vi "FeedbackDecode.vi"() -> ()   [LabVIEW 2020] (continued)
                n1302 = local read "NIPTime"() -> (w1168:dbl)
                n1303 = Concatenate Strings(w1160, w1180, w1179, w1178) -> (w1186:string)
                n1304 = Concatenate Strings("AutoPop:SS.EventID=" ("string"), w1164) -> (w1172:string)
                n1305 = local read "EventParamsFID"() -> (w1171:refnum<file>)
                n1306 = call-poly "FeedbackDecode_VariablesToString.vi"("Format"="%0.0f", "ValueIn"=w1168, "FieldName"="NIPTime" ("Key Word")) -> ("StringOut"=w1165:string)  [unwired: 4 in]
                n1307 = Concatenate Strings(w1172, ";", w1186, w1165) -> (w1170:string)
                n1308 = call "FeedbackDecode_WriteTextEOL.vi"("text"=w1170, "refnum in"=w1171) -> ()  [unwired: 8 in, 2 out]
                n1309 = Bundle By Name(cluster=w1187, "EventStr"=w1170) -> (w1169:T5)
                n1310 = call "FeedbackDecode_MLComCtrl.vi"("DecodeClustIn"=w1169, "Mode"=T19."SendEvent") -> ()  [unwired: 6 in, 4 out]
              }
            }
          }
          event Value Change {
            n1311 = event-data() -> ()  [unwired: 1 in, 6 out]
            n1312 = local read "DecodeClust"() -> (w1208:T5)
            n1313 = Unbundle By Name(w1208) -> ("BadUEAElects"=w1200:dbl[], "BadEMGChans"=w1203:dbl[])
            n1314 = local read "LoopCnt"() -> (w1196:u64)
            n1315 = call-poly "FeedbackDecode_VariablesToString.vi"("ValueIn"=w1200, "FieldName"="BadUEAElects") -> ("StringOut"=w1202:string)  [unwired: 5 in]
            n1316 = call-poly "FeedbackDecode_VariablesToString.vi"("ValueIn"=w1203, "FieldName"="BadEMGChans") -> ("StringOut"=w1201:string)  [unwired: 5 in]
            n1317 = Format Into String(w1196) -> (resulting string=w1188:string)  [unwired: 3 in, 1 out]
            n1318 = local read "NIPTime"() -> (w1192:dbl)
            n1319 = Concatenate Strings(w1202, w1201) -> (w1206:string)
            n1320 = Concatenate Strings("SendBad:SS.EventID=" ("string"), w1188) -> (w1195:string)
            n1321 = local read "EventParamsFID"() -> (w1207:refnum<file>)
            n1322 = call-poly "FeedbackDecode_VariablesToString.vi"("Format"="%0.0f", "ValueIn"=w1192, "FieldName"="NIPTime" ("Key Word")) -> ("StringOut"=w1189:string)  [unwired: 4 in]
            n1323 = Concatenate Strings(w1195, ";", w1206, w1189) -> (w1194:string)
            n1324 = call "FeedbackDecode_WriteTextEOL.vi"("text"=w1194, "refnum in"=w1207) -> ()  [unwired: 8 in, 2 out]
            n1325 = Bundle By Name(cluster=w1208, "EventStr"=w1194) -> (w1193:T5)
            n1326 = call "FeedbackDecode_MLComCtrl.vi"("DecodeClustIn"=w1193, "Mode"=T19."SendEvent") -> ()  [unwired: 6 in, 4 out]
          }
          event Value Change {
            n1327 = event-data() -> ("NewVal"=w1212:bool)  [unwired: 1 in, 5 out]
            n1328 = Not(x=w1212) -> (.not. x?=w1211:bool)
            n1329 = local read "DecodeClust"() -> (w1213:T5)
            n1330 = Bundle By Name(cluster=w1213, "CtrlButtons.Stop"=w1211) -> (w1210:T5)
            n1331 = local write "DecodeClust"(w1210) -> ()
            n1332 = property on="Finished" class="Bool (strict)"("DisabledEnum"=T17."Enabled" ("Disabled"), "Blinking"=TRUE) -> ()  [unwired: 2 in, 2 out]
            n1333 = local write "LVTab"(enum32{"Decode", "Encode", "Video", "Database"}."Database" ("LVTab")) -> ()
          }
          event "Finished": Value Change {
            n1334 = event-data() -> ("NewVal"=w1218:bool)  [unwired: 1 in, 5 out]
            n1335 = global write "FeedbackDecode_Globals.vi" "FD_Stop"(w1218) -> ()
          }
          event Value Change {
            n1336 = event-data() -> ("NewVal"=w1219:bool)  [unwired: 1 in, 5 out]
            n1337 = case shown="True" w1219 {
              frame False {
                n1338 = local read "LoopCnt"() -> (w1229:u64)
                n1339 = local read "NIPTime"() -> (w1225:dbl)
                n1340 = Format Into String(w1229) -> (resulting string=w1221:string)  [unwired: 3 in, 1 out]
                n1341 = local read "EventParamsFID"() -> (w1233:refnum<file>)
                n1342 = local read "DecodeClust"() -> (w1234:T5)
                n1343 = call-poly "FeedbackDecode_VariablesToString.vi"("Format"="%0.0f", "ValueIn"=w1225, "FieldName"="NIPTime" ("Key Word")) -> ("StringOut"=w1222:string)  [unwired: 4 in]
                n1344 = Concatenate Strings("DisableStartTrials:SS.EventID=" ("string"), w1221) -> (w1228:string)
                n1345 = Concatenate Strings(w1228, ";", w1222) -> (w1227:string)
                n1346 = call "FeedbackDecode_WriteTextEOL.vi"("text"=w1227, "refnum in"=w1233) -> ()  [unwired: 8 in, 2 out]
                n1347 = Bundle By Name(cluster=w1234, "EventStr"=w1227) -> (w1226:T5)
                n1348 = call "FeedbackDecode_MLComCtrl.vi"("DecodeClustIn"=w1226, "Mode"=T19."SendEvent") -> ()  [unwired: 6 in, 4 out]
              }
              frame True {
                n1349 = local read "LoopCnt"() -> (w1248:u64)
                n1350 = local read "NIPTime"() -> (w1239:dbl)
                n1351 = Format Into String(w1248) -> (resulting string=w1235:string)  [unwired: 3 in, 1 out]
                n1352 = local read "EventParamsFID"() -> (w1252:refnum<file>)
                n1353 = call-poly "FeedbackDecode_VariablesToString.vi"("Format"="%0.0f", "ValueIn"=w1239, "FieldName"="NIPTime" ("Key Word")) -> ("StringOut"=w1236:string)  [unwired: 4 in]
                n1354 = Concatenate Strings("EnableStartTrials:SS.EventID=" ("string"), w1235) -> (w1247:string)
                n1355 = Concatenate Strings(w1247, ";", w1236) -> (w1246:string)
                n1356 = local read "DecodeClust"() -> (w1253:T5)
                n1357 = call "FeedbackDecode_WriteTextEOL.vi"("text"=w1246, "refnum in"=w1252) -> ()  [unwired: 8 in, 2 out]
                n1358 = Initialize Array(0.0 ("element"), 2 ("dimension size"), 12 ("dimension size")) -> (w1241:dbl[][])
                n1359 = Bundle By Name(cluster=w1253, "EventStr"=w1246, "TrialCnt"=w1241) -> (w1245:T5)
                n1360 = local read "LoopCnt"() -> (w1255:u64)
                n1361 = local write "ResetCorr"(TRUE ("ResetCorr")) -> ()
                n1362 = call "FeedbackDecode_MLComCtrl.vi"("DecodeClustIn"=w1245, "Mode"=T19."SendEvent") -> ("DecodeClustOut"=w1240:T5)  [unwired: 6 in, 3 out]
                n1363 = local write "BaseCnt1"(w1255) -> ()
                n1364 = local write "DecodeClust"(w1240) -> ()
              }
            }
          }
          event Value Change {
            n1365 = event-data() -> ("CtlRef"=w1267:refnum<vi>)  [unwired: 1 in, 5 out]
            n1366 = property class="Ctl"(reference=w1267) -> ("Label.Text"=w1266:string)  [unwired: 1 in, 2 out]
            n1367 = case shown="\"ResetTrial\"" w1266 {
              frame "", Default {
              }
              frame "ResetTrial" {
                n1368 = local read "State"() -> (w1269:T16)
                n1369 = case shown="\"Acquire Start\", Default" w1269 {
                  frame "Initialize" {
                    n1370 = local read "DecodeClust"() -> (w1272:T5)
                    n1371 = Bundle By Name(cluster=w1272, "CtrlButtons.ResetTrial"=FALSE) -> (w1271:T5)
                    n1372 = local write "DecodeClust"(w1271) -> ()
                  }
                  frame "Acquire Start", Default {
                    n1373 = local read "NIPTime"() -> (w1277:dbl)
                    n1374 = local read "LoopCnt"() -> (w1281:u64)
                    n1375 = call-poly "FeedbackDecode_VariablesToString.vi"("Format"="%0.0f", "ValueIn"=w1277, "FieldName"="NIPTime" ("Key Word")) -> ("StringOut"=w1274:string)  [unwired: 4 in]
                    n1376 = Format Into String(w1281) -> (resulting string=w1273:string)  [unwired: 3 in, 1 out]
                    n1377 = local read "EventParamsFID"() -> (w1285:refnum<file>)
                    n1378 = local read "DecodeClust"() -> (w1286:T5)
                    n1379 = Concatenate Strings("ResetTrial:SS.EventID=" ("string"), w1273) -> (w1280:string)
                    n1380 = Concatenate Strings(w1280, ";", w1274) -> (w1279:string)
                    n1381 = call "FeedbackDecode_WriteTextEOL.vi"("text"=w1279, "refnum in"=w1285) -> ()  [unwired: 8 in, 2 out]
                    n1382 = Bundle By Name(cluster=w1286, "EventStr"=w1279) -> (w1278:T5)
                    n1383 = call "FeedbackDecode_MLComCtrl.vi"("DecodeClustIn"=w1278, "Mode"=T19."SendEvent") -> ()  [unwired: 6 in, 4 out]
                  }
                }
              }
            }
            n1384 = local read "MvntBuilder"() -> (w1258:T6)
            n1385 = Unbundle By Name(w1258) -> ("Mode"=w1265:enum16{"Selected", "Block", "Random"}, "NTrials"=w1262:dbl, "MvntList"=w1261:T24)
            n1386 = property on="MvntList" class="Arr (strict)"() -> ("Index Values"=w1259:u32[])  [unwired: 2 in, 2 out]
            n1387 = Array Size(array=w1261) -> (size(s)=w1260:i32)
            n1388 = Index Array(array=w1259) -> (element=w1263:u32)  [unwired: 1 in]
            n1389 = call "FeedbackDecode_GenRandBlockIdxs2.vi"("Mode"=w1265, "Reset"=TRUE, "NumTrials"=w1262, "NumIdxs"=w1260, "CurrIdx"=w1263) -> ("Perc"=w1257:dbl)  [unwired: 1 out]
            n1390 = Bundle By Name(cluster=w1258, "PercTrials"=w1257) -> (w1256:T6)
            n1391 = local write "MvntBuilder"(w1256) -> ()
          }
          event Value Change {
            n1392 = event-data() -> ("NewVal"=w1287:bool)  [unwired: 1 in, 5 out]
            n1393 = case shown="True" w1287 {
              frame False {
                n1394 = local read "LoopCnt"() -> (w1299:u64)
                n1395 = local read "NIPTime"() -> (w1293:dbl)
                n1396 = Format Into String(w1299) -> (resulting string=w1289:string)  [unwired: 3 in, 1 out]
                n1397 = call-poly "FeedbackDecode_VariablesToString.vi"("Format"="%0.0f", "ValueIn"=w1293, "FieldName"="NIPTime" ("Key Word")) -> ("StringOut"=w1290:string)  [unwired: 4 in]
                n1398 = Concatenate Strings("DisableHideSpheres:SS.EventID=" ("string"), w1289) -> (w1298:string)
                n1399 = local read "EventParamsFID"() -> (w1296:refnum<file>)
                n1400 = local read "DecodeClust"() -> (w1302:T5)
                n1401 = Concatenate Strings(w1298, ";SS.HideSpheres=0;" ("EventStr"), w1290) -> (w1295:string)
                n1402 = call "FeedbackDecode_WriteTextEOL.vi"("text"=w1295, "refnum in"=w1296) -> ()  [unwired: 8 in, 2 out]
                n1403 = Bundle By Name(cluster=w1302, "EventStr"=w1295) -> (w1294:T5)
                n1404 = call "FeedbackDecode_MLComCtrl.vi"("DecodeClustIn"=w1294, "Mode"=T19."SendEvent") -> ()  [unwired: 6 in, 4 out]
              }
              frame True {
                n1405 = local read "LoopCnt"() -> (w1313:u64)
                n1406 = local read "NIPTime"() -> (w1307:dbl)
                n1407 = Format Into String(w1313) -> (resulting string=w1303:string)  [unwired: 3 in, 1 out]
                n1408 = Concatenate Strings("EnableHideSpheres:SS.EventID=" ("string"), w1303) -> (w1312:string)
                n1409 = call-poly "FeedbackDecode_VariablesToString.vi"("Format"="%0.0f", "ValueIn"=w1307, "FieldName"="NIPTime" ("Key Word")) -> ("StringOut"=w1304:string)  [unwired: 4 in]
                n1410 = local read "EventParamsFID"() -> (w1310:refnum<file>)
                n1411 = local read "DecodeClust"() -> (w1316:T5)
                n1412 = Concatenate Strings(w1312, ";SS.HideSpheres=1;" ("EventStr"), w1304) -> (w1309:string)
                n1413 = call "FeedbackDecode_WriteTextEOL.vi"("text"=w1309, "refnum in"=w1310) -> ()  [unwired: 8 in, 2 out]
                n1414 = Bundle By Name(cluster=w1316, "EventStr"=w1309) -> (w1308:T5)
                n1415 = call "FeedbackDecode_MLComCtrl.vi"("DecodeClustIn"=w1308, "Mode"=T19."SendEvent") -> ()  [unwired: 6 in, 4 out]
              }
            }
          }
          event Value Change {
            n1416 = event-data() -> ("NewVal"=w1318:T44)  [unwired: 1 in, 5 out]
            n1417 = Format Into String(w1318) -> (resulting string=w1317:string)  [unwired: 3 in, 1 out]
            n1418 = local read "LoopCnt"() -> (w1327:u64)
            n1419 = call-poly "FeedbackDecode_VariablesToString.vi"("ValueIn"=w1317, "FieldName"="KalmanType") -> ("StringOut"=w1334:string)  [unwired: 5 in]
            n1420 = local read "NIPTime"() -> (w1323:dbl)
            n1421 = Format Into String(w1327) -> (resulting string=w1319:string)  [unwired: 3 in, 1 out]
            n1422 = local read "EventParamsFID"() -> (w1331:refnum<file>)
            n1423 = local read "DecodeClust"() -> (w1332:T5)
            n1424 = Concatenate Strings("ChangeKalmanType:SS.EventID=" ("string"), w1319) -> (w1326:string)
            n1425 = call-poly "FeedbackDecode_VariablesToString.vi"("Format"="%0.0f", "ValueIn"=w1323, "FieldName"="NIPTime" ("Key Word")) -> ("StringOut"=w1320:string)  [unwired: 4 in]
            n1426 = Concatenate Strings(w1326, ";", w1334, w1320) -> (w1325:string)
            n1427 = call "FeedbackDecode_WriteTextEOL.vi"("text"=w1325, "refnum in"=w1331) -> ()  [unwired: 8 in, 2 out]
            n1428 = Bundle By Name(cluster=w1332, "EventStr"=w1325) -> (w1324:T5)
            n1429 = call "FeedbackDecode_MLComCtrl.vi"("DecodeClustIn"=w1324, "Mode"=T19."SendEvent") -> ()  [unwired: 6 in, 4 out]
          }
          event Value Change {
            n1430 = event-data() -> ()  [unwired: 1 in, 6 out]
            n1431 = call "Load NN"("prompt"="select a .mat file that contains the trained NN") -> ("selected path"=w1338:path)  [unwired: 11 in, 3 out]
            n1432 = Path To String(path=w1338) -> (string=w1337:string)
            n1433 = local read "LoopCnt"() -> (w1347:u64)
            n1434 = call-poly "FeedbackDecode_VariablesToString.vi"("ValueIn"=w1337, "FieldName"="NN.path") -> ("StringOut"=w1354:string)  [unwired: 5 in]
            n1435 = local read "NIPTime"() -> (w1343:dbl)
            n1436 = Format Into String(w1347) -> (resulting string=w1339:string)  [unwired: 3 in, 1 out]
            n1437 = local read "EventParamsFID"() -> (w1351:refnum<file>)
            n1438 = Concatenate Strings("LoadNN:SS.EventID=" ("string"), w1339) -> (w1346:string)
            n1439 = call-poly "FeedbackDecode_VariablesToString.vi"("Format"="%0.0f", "ValueIn"=w1343, "FieldName"="NIPTime" ("Key Word")) -> ("StringOut"=w1340:string)  [unwired: 4 in]
            n1440 = Concatenate Strings(w1346, ";", w1354, w1340) -> (w1345:string)
            n1441 = local read "DecodeClust"() -> (w1352:T5)
            n1442 = call "FeedbackDecode_WriteTextEOL.vi"("text"=w1345, "refnum in"=w1351) -> ()  [unwired: 8 in, 2 out]
            n1443 = Bundle By Name(cluster=w1352, "EventStr"=w1345) -> (w1344:T5)
            n1444 = call "FeedbackDecode_MLComCtrl.vi"("DecodeClustIn"=w1344, "Mode"=T19."SendEvent") -> ()  [unwired: 6 in, 4 out]
          }
          event "CalibrateTASKA": Value Change {
            n1445 = event-data() -> ()  [unwired: 1 in, 6 out]
            n1446 = local read "LoopCnt"() -> (w1364:u64)
            n1447 = local read "NIPTime"() -> (w1360:dbl)
            n1448 = Format Into String(w1364) -> (resulting string=w1356:string)  [unwired: 3 in, 1 out]
            n1449 = local read "EventParamsFID"() -> (w1368:refnum<file>)
            n1450 = Concatenate Strings("CalibrateTASKA:SS.EventID=" ("string"), w1356) -> (w1363:string)
            n1451 = call-poly "FeedbackDecode_VariablesToString.vi"("Format"="%0.0f", "ValueIn"=w1360, "FieldName"="NIPTime" ("Key Word")) -> ("StringOut"=w1357:string)  [unwired: 4 in]
            n1452 = Concatenate Strings(w1363, ";", w1357) -> (w1362:string)
            n1453 = local read "DecodeClust"() -> (w1369:T5)
            n1454 = call "FeedbackDecode_WriteTextEOL.vi"("text"=w1362, "refnum in"=w1368) -> ()  [unwired: 8 in, 2 out]
            n1455 = Bundle By Name(cluster=w1369, "EventStr"=w1362) -> (w1361:T5)
            n1456 = call "FeedbackDecode_MLComCtrl.vi"("DecodeClustIn"=w1361, "Mode"=T19."SendEvent") -> ()  [unwired: 6 in, 4 out]
          }
          event "Reset Calibration": Value Change {
            n1457 = event-data() -> ()  [unwired: 1 in, 6 out]
            n1458 = local read "LoopCnt"() -> (w1379:u64)
            n1459 = local read "NIPTime"() -> (w1375:dbl)
            n1460 = Format Into String(w1379) -> (resulting string=w1371:string)  [unwired: 3 in, 1 out]
            n1461 = local read "EventParamsFID"() -> (w1383:refnum<file>)
            n1462 = Concatenate Strings("CalibrateTASKAreset:SS.EventID=" ("string"), w1371) -> (w1378:string)
            n1463 = call-poly "FeedbackDecode_VariablesToString.vi"("Format"="%0.0f", "ValueIn"=w1375, "FieldName"="NIPTime" ("Key Word")) -> ("StringOut"=w1372:string)  [unwired: 4 in]
            n1464 = Concatenate Strings(w1378, ";", w1372) -> (w1377:string)
            n1465 = local read "DecodeClust"() -> (w1384:T5)
            n1466 = call "FeedbackDecode_WriteTextEOL.vi"("text"=w1377, "refnum in"=w1383) -> ()  [unwired: 8 in, 2 out]
            n1467 = Bundle By Name(cluster=w1384, "EventStr"=w1377) -> (w1376:T5)
            n1468 = call "FeedbackDecode_MLComCtrl.vi"("DecodeClustIn"=w1376, "Mode"=T19."SendEvent") -> ()  [unwired: 6 in, 4 out]
          }
          event "LoadCyberGlove": Value Change {
            n1469 = event-data() -> ()  [unwired: 1 in, 6 out]
            n1470 = call "Load NN2"("prompt"="select a .mat file that contains the cyberglove calibration") -> ("selected path"=w1388:path)  [unwired: 11 in, 3 out]
            n1471 = Path To String(path=w1388) -> (string=w1387:string)
            n1472 = local read "LoopCnt"() -> (w1397:u64)
            n1473 = call-poly "FeedbackDecode_VariablesToString.vi"("ValueIn"=w1387, "FieldName"="CyberGlove.Calibration") -> ("StringOut"=w1404:string)  [unwired: 5 in]
            n1474 = local read "NIPTime"() -> (w1393:dbl)
            n1475 = Format Into String(w1397) -> (resulting string=w1389:string)  [unwired: 3 in, 1 out]
            n1476 = local read "EventParamsFID"() -> (w1401:refnum<file>)
            n1477 = local read "DecodeClust"() -> (w1402:T5)
            n1478 = Concatenate Strings("LoadCyberGlove:SS.EventID=" ("string"), w1389) -> (w1396:string)
            n1479 = call-poly "FeedbackDecode_VariablesToString.vi"("Format"="%0.0f", "ValueIn"=w1393, "FieldName"="NIPTime" ("Key Word")) -> ("StringOut"=w1390:string)  [unwired: 4 in]
            n1480 = Concatenate Strings(w1396, ";", w1404, w1390) -> (w1395:string)
            n1481 = call "FeedbackDecode_WriteTextEOL.vi"("text"=w1395, "refnum in"=w1401) -> ()  [unwired: 8 in, 2 out]
            n1482 = Bundle By Name(cluster=w1402, "EventStr"=w1395) -> (w1394:T5)
            n1483 = call "FeedbackDecode_MLComCtrl.vi"("DecodeClustIn"=w1394, "Mode"=T19."SendEvent") -> ()  [unwired: 6 in, 4 out]
          }
          event "Stim Thresholds": Value Change {
            # "convert from Newtons to 0 to 1 sensor value"
            n1484 = event-data() -> ("NewVal"=w1408:dbl[])  [unwired: 1 in, 5 out]
            n1485 = Divide(x=w1408, y=25.5) -> (x/y=w1409:dbl[])
            n1486 = local read "LoopCnt"() -> (w1418:u64)
            n1487 = call-poly "FeedbackDecode_VariablesToString.vi"("Format"="%0.6f", "ValueIn"=w1409, "FieldName"="DEKA.SensorThresholds") -> ("StringOut"=w1425:string)  [unwired: 4 in]
            n1488 = local read "NIPTime"() -> (w1414:dbl)
            n1489 = Format Into String(w1418) -> (resulting string=w1410:string)  [unwired: 3 in, 1 out]
            n1490 = local read "EventParamsFID"() -> (w1422:refnum<file>)
            n1491 = local read "DecodeClust"() -> (w1423:T5)
            n1492 = Concatenate Strings("UpdateSensorThresholds:SS.EventID=" ("string"), w1410) -> (w1417:string)
            n1493 = call-poly "FeedbackDecode_VariablesToString.vi"("Format"="%0.0f", "ValueIn"=w1414, "FieldName"="NIPTime" ("Key Word")) -> ("StringOut"=w1411:string)  [unwired: 4 in]
            n1494 = Concatenate Strings(w1417, ";", w1425, w1411) -> (w1416:string)
            n1495 = call "FeedbackDecode_WriteTextEOL.vi"("text"=w1416, "refnum in"=w1422) -> ()  [unwired: 8 in, 2 out]
            n1496 = Bundle By Name(cluster=w1423, "EventStr"=w1416) -> (w1415:T5)
            n1497 = call "FeedbackDecode_MLComCtrl.vi"("DecodeClustIn"=w1415, "Mode"=T19."SendEvent") -> ()  [unwired: 6 in, 4 out]
          }
          event Value Change {
            n1498 = event-data() -> ("NewVal"=w1433:string)  [unwired: 1 in, 5 out]
            n1499 = local read "LoopCnt"() -> (w1436:u64)
            n1500 = local read "NIPTime"() -> (w1431:dbl)
            n1501 = Format Into String(w1436) -> (resulting string=w1427:string)  [unwired: 3 in, 1 out]
            n1502 = local read "DecodeClust"() -> (w1441:T5)
            n1503 = Concatenate Strings("SS.LinkedDOF=" ("FieldName"), w1433, ";" ("string")) -> (w1444:string)
            n1504 = local read "EventParamsFID"() -> (w1440:refnum<file>)
            n1505 = Concatenate Strings("LinkDOF:SS.EventID=" ("string"), w1427) -> (w1435:string)
            n1506 = call-poly "FeedbackDecode_VariablesToString.vi"("Format"="%0.0f", "ValueIn"=w1431, "FieldName"="NIPTime" ("Key Word")) -> ("StringOut"=w1428:string)  [unwired: 4 in]
            n1507 = Concatenate Strings(w1435, ";", w1444, w1428) -> (w1434:string)
            n1508 = call "FeedbackDecode_WriteTextEOL.vi"("text"=w1434, "refnum in"=w1440) -> ()  [unwired: 8 in, 2 out]
            n1509 = Bundle By Name(cluster=w1441, "EventStr"=w1434) -> (w1432:T5)
            n1510 = call "FeedbackDecode_MLComCtrl.vi"("DecodeClustIn"=w1432, "Mode"=T19."SendEvent") -> ()  [unwired: 6 in, 4 out]
          }
          event Value Change {
            n1511 = event-data() -> ("NewVal"=w1452:enum16{"Standard", "Stepwise", "Gram"})  [unwired: 1 in, 5 out]
            n1512 = local read "LoopCnt"() -> (w1455:u64)
            n1513 = call-poly "FeedbackDecode_VariablesToString.vi"("Format"="%0.0f", "ValueIn"=w1452, "FieldName"="AutoPopType") -> ("StringOut"=w1463:string)  [unwired: 4 in]
            n1514 = local read "NIPTime"() -> (w1450:dbl)
            n1515 = Format Into String(w1455) -> (resulting string=w1446:string)  [unwired: 3 in, 1 out]
            n1516 = local read "EventParamsFID"() -> (w1459:refnum<file>)
            n1517 = local read "DecodeClust"() -> (w1460:T5)
            n1518 = Concatenate Strings("ChangeAutoPopType:SS.EventID=" ("string"), w1446) -> (w1454:string)
            n1519 = call-poly "FeedbackDecode_VariablesToString.vi"("Format"="%0.0f", "ValueIn"=w1450, "FieldName"="NIPTime" ("Key Word")) -> ("StringOut"=w1447:string)  [unwired: 4 in]
            n1520 = Concatenate Strings(w1454, ";", w1463, w1447) -> (w1453:string)
            n1521 = call "FeedbackDecode_WriteTextEOL.vi"("text"=w1453, "refnum in"=w1459) -> ()  [unwired: 8 in, 2 out]
            n1522 = Bundle By Name(cluster=w1460, "EventStr"=w1453) -> (w1451:T5)
            n1523 = call "FeedbackDecode_MLComCtrl.vi"("DecodeClustIn"=w1451, "Mode"=T19."SendEvent") -> ()  [unwired: 6 in, 4 out]
          }
          event Value Change {
            n1524 = event-data() -> ("NewVal"=w1466:enum16{"Standard", "NN"})  [unwired: 1 in, 5 out]
            n1525 = Format Into String(w1466) -> (resulting string=w1465:string)  [unwired: 3 in, 1 out]
            n1526 = local read "LoopCnt"() -> (w1475:u64)
            n1527 = call-poly "FeedbackDecode_VariablesToString.vi"("ValueIn"=w1465, "FieldName"="CARType") -> ("StringOut"=w1482:string)  [unwired: 5 in]
            n1528 = local read "NIPTime"() -> (w1471:dbl)
            n1529 = Format Into String(w1475) -> (resulting string=w1467:string)  [unwired: 3 in, 1 out]
            n1530 = local read "EventParamsFID"() -> (w1479:refnum<file>)
            n1531 = Concatenate Strings("ChangeCARType:SS.EventID=" ("string"), w1467) -> (w1474:string)
            n1532 = local read "DecodeClust"() -> (w1480:T5)
            n1533 = call-poly "FeedbackDecode_VariablesToString.vi"("Format"="%0.0f", "ValueIn"=w1471, "FieldName"="NIPTime" ("Key Word")) -> ("StringOut"=w1468:string)  [unwired: 4 in]
            n1534 = Concatenate Strings(w1474, ";", w1482, w1468) -> (w1473:string)
            n1535 = call "FeedbackDecode_WriteTextEOL.vi"("text"=w1473, "refnum in"=w1479) -> ()  [unwired: 8 in, 2 out]
            n1536 = Bundle By Name(cluster=w1480, "EventStr"=w1473) -> (w1472:T5)
            n1537 = call "FeedbackDecode_MLComCtrl.vi"("DecodeClustIn"=w1472, "Mode"=T19."SendEvent") -> ()  [unwired: 6 in, 4 out]
          }
          event Value Change {
            n1538 = event-data() -> ("NewVal"=w1486:bool)  [unwired: 1 in, 5 out]
            n1539 = Boolean To (0,1)(Boolean=w1486) -> (0, 1=w1485:i16)
            n1540 = local read "LoopCnt"() -> (w1495:u64)
            n1541 = call-poly "FeedbackDecode_VariablesToString.vi"("Format"="%0.0f", "ValueIn"=w1485, "FieldName"="LimitExt") -> ("StringOut"=w1502:string)  [unwired: 4 in]
            n1542 = local read "NIPTime"() -> (w1491:dbl)
            n1543 = Format Into String(w1495) -> (resulting string=w1487:string)  [unwired: 3 in, 1 out]
            n1544 = local read "DecodeClust"() -> (w1500:T5)
            n1545 = local read "EventParamsFID"() -> (w1499:refnum<file>)
            n1546 = Concatenate Strings("LimitExt:SS.EventID=" ("string"), w1487) -> (w1494:string)
            n1547 = call-poly "FeedbackDecode_VariablesToString.vi"("Format"="%0.0f", "ValueIn"=w1491, "FieldName"="NIPTime" ("Key Word")) -> ("StringOut"=w1488:string)  [unwired: 4 in]
            n1548 = Concatenate Strings(w1494, ";", w1502, w1488) -> (w1493:string)
            n1549 = call "FeedbackDecode_WriteTextEOL.vi"("text"=w1493, "refnum in"=w1499) -> ()  [unwired: 8 in, 2 out]
            n1550 = Bundle By Name(cluster=w1500, "EventStr"=w1493) -> (w1492:T5)
            n1551 = call "FeedbackDecode_MLComCtrl.vi"("DecodeClustIn"=w1492, "Mode"=T19."SendEvent") -> ()  [unwired: 6 in, 4 out]
          }
          event Value Change {
            n1552 = event-data() -> ("NewVal"=w1506:bool)  [unwired: 1 in, 5 out]
            n1553 = Boolean To (0,1)(Boolean=w1506) -> (0, 1=w1505:i16)
            n1554 = local read "LoopCnt"() -> (w1515:u64)
            n1555 = call-poly "FeedbackDecode_VariablesToString.vi"("Format"="%0.0f", "ValueIn"=w1505, "FieldName"="DynFlag") -> ("StringOut"=w1522:string)  [unwired: 4 in]
            n1556 = local read "NIPTime"() -> (w1511:dbl)
            n1557 = Format Into String(w1515) -> (resulting string=w1507:string)  [unwired: 3 in, 1 out]
            n1558 = local read "DecodeClust"() -> (w1520:T5)
            n1559 = local read "EventParamsFID"() -> (w1519:refnum<file>)
            n1560 = Concatenate Strings("DynFlag:SS.EventID=" ("string"), w1507) -> (w1514:string)
            n1561 = call-poly "FeedbackDecode_VariablesToString.vi"("Format"="%0.0f", "ValueIn"=w1511, "FieldName"="NIPTime" ("Key Word")) -> ("StringOut"=w1508:string)  [unwired: 4 in]
            n1562 = Concatenate Strings(w1514, ";", w1522, w1508) -> (w1513:string)
            n1563 = call "FeedbackDecode_WriteTextEOL.vi"("text"=w1513, "refnum in"=w1519) -> ()  [unwired: 8 in, 2 out]
            n1564 = Bundle By Name(cluster=w1520, "EventStr"=w1513) -> (w1512:T5)
            n1565 = call "FeedbackDecode_MLComCtrl.vi"("DecodeClustIn"=w1512, "Mode"=T19."SendEvent") -> ()  [unwired: 6 in, 4 out]
          }
          event Mouse Move {
            n1566 = event-data() -> ("Coords"=w1531:T45)  [unwired: 1 in, 3 out]
            n1567 = local read "HoverPicPos"() -> (w1529:T14)
            n1568 = call "FeedbackDecode_HoverElect.vi"("Border"=2.0, "PicPos"=w1529, "MousePos"=w1531, "Mode"=enum16{"Initialize", "Run"}."Run") -> ("Elect"=w1524:i32)  [unwired: 2 in, 1 out]
            n1569 = local read "DecodeClust"() -> (w1526:T5)
            n1570 = Bundle By Name(cluster=w1526, "HoverElect"=w1524) -> (w1525:T5)
            n1571 = local write "DecodeClust"(w1525) -> ()
          }
          event Value Change {
            # "Also updated CtrlMode and CtrlSpd"
            n1572 = event-data() -> ()  [unwired: 1 in, 6 out]
            n1573 = local read "DecodeClust"() -> (w1537:T5)
            n1574 = Unbundle By Name(w1537) -> ("KMvntClust"=w1538:T46)
            n1575 = call "FeedbackDecode_KalmanMvnts2Str.vi"("KMvntClust"=w1538) -> ("KMvntStr"=w1534:string)
            n1576 = Concatenate Strings("UpdateKGainThresh:" ("string"), w1534) -> (w1533:string)
            n1577 = Bundle By Name(cluster=w1537, "EventStr"=w1533) -> (w1532:T5)
            n1578 = call "FeedbackDecode_MLComCtrl.vi"("DecodeClustIn"=w1532, "Mode"=T19."SendEvent") -> ()  [unwired: 6 in, 4 out]
          }
          event Value Change {
            n1579 = event-data() -> ("NewVal"=w1541:bool)  [unwired: 1 in, 5 out]
            n1580 = case shown="True" w1541 {
              frame False {
              }
              frame True {
                n1581 = local read "DecodeClust"() -> (w1565:T5)
                n1582 = Unbundle By Name(w1565) -> ("ThreshMode"=w1543:T47, "ThreshVal"=w1560:dbl)
                n1583 = Format Into String(w1543) -> (resulting string=w1542:string)  [unwired: 3 in, 1 out]
                n1584 = local read "LoopCnt"() -> (w1554:u64)
                n1585 = call-poly "FeedbackDecode_VariablesToString.vi"("ValueIn"=w1542, "FieldName"="ThreshMode") -> ("StringOut"=w1562:string)  [unwired: 5 in]
                n1586 = call-poly "FeedbackDecode_VariablesToString.vi"("ValueIn"=w1560, "FieldName"="ThreshVal") -> ("StringOut"=w1559:string)  [unwired: 5 in]
                n1587 = local read "NIPTime"() -> (w1548:dbl)
                n1588 = Concatenate Strings(w1562, w1559) -> (w1564:string)
                n1589 = Format Into String(w1554) -> (resulting string=w1544:string)  [unwired: 3 in, 1 out]
                n1590 = local read "EventParamsFID"() -> (w1558:refnum<file>)
                n1591 = call-poly "FeedbackDecode_VariablesToString.vi"("Format"="%0.0f", "ValueIn"=w1548, "FieldName"="NIPTime" ("Key Word")) -> ("StringOut"=w1545:string)  [unwired: 4 in]
                n1592 = Concatenate Strings("UpdateThresh:SS.EventID=" ("string"), w1544) -> (w1553:string)
                n1593 = Concatenate Strings(w1553, ";", w1564, w1545) -> (w1552:string)
                n1594 = call "FeedbackDecode_WriteTextEOL.vi"("text"=w1552, "refnum in"=w1558) -> ()  [unwired: 8 in, 2 out]
                n1595 = Bundle By Name(cluster=w1565, "EventStr"=w1552, "ApplyThresh"=FALSE) -> (w1551:T5)
                n1596 = call "FeedbackDecode_MLComCtrl.vi"("DecodeClustIn"=w1551, "Mode"=T19."SendEvent") -> ("DecodeClustOut"=w1549:T5)  [unwired: 6 in, 3 out]
                n1597 = local write "DecodeClust"(w1549) -> ()
              }
            }
          }
          event Value Change {
            n1598 = event-data() -> ("NewVal"=w1570:dbl)  [unwired: 1 in, 5 out]
            n1599 = Divide(x=w1570, y=0.033) -> (x/y=w1566:dbl)
            n1600 = Multiply(x=2.0, y=w1566) -> (x*y=w1568:dbl)
            n1601 = property on="SelData" class="WFGraph (strict)"("XScale.Maximum"=w1568) -> ()  [unwired: 2 in, 2 out]
            n1602 = property on="SelRate" class="WFGraph (strict)"("XScale.Maximum"=w1566) -> ()  [unwired: 2 in, 2 out]
            n1603 = property on="SelKin" class="WFGraph (strict)"("XScale.Maximum"=w1566) -> ()  [unwired: 2 in, 2 out]
          }
          event Value Change {
            n1604 = event-data() -> ("NewVal"=w1573:bool)  [unwired: 1 in, 5 out]
            n1605 = case shown="True" w1573 {
              frame False {
              }
              frame True {
                n1606 = for {
                  N: 2 -> [_]
                  tunnel: [w1579] -> w1574 mode=indexing
                  n1607 = Initialize Array(FALSE, 100 ("dimension size")) -> (w1580:bool[])
                  n1608 = Array To Cluster(array=w1580) -> (cluster=w1579:T48)
                }
                n1609 = local read "DecodeClust"() -> (w1577:T5)
                n1610 = Bundle By Name(cluster=w1577, "ClearUEA"=FALSE ("CtrlButtons.ResetTrial"), "KUEAArray"=w1574) -> (w1576:T5)
                n1611 = local write "DecodeClust"(w1576) -> ()
              }
            }
          }
          event Value Change {
            n1612 = event-data() -> ("NewVal"=w1584:bool)  [unwired: 1 in, 5 out]
            n1613 = case shown="True" w1584 {
              frame False {
              }
              frame True {
                n1614 = for {
                  N: 2 -> [_]
                  tunnel: [w1590] -> w1585 mode=indexing
                  n1615 = Initialize Array(TRUE, 100 ("dimension size")) -> (w1591:bool[])
                  n1616 = Array To Cluster(array=w1591) -> (cluster=w1590:T48)
                }
                n1617 = local read "DecodeClust"() -> (w1588:T5)
                n1618 = Bundle By Name(cluster=w1588, "FillUEA"=FALSE ("CtrlButtons.ResetTrial"), "KUEAArray"=w1585) -> (w1587:T5)
                n1619 = local write "DecodeClust"(w1587) -> ()
              }
            }
          }
          event Value Change {
            n1620 = event-data() -> ("NewVal"=w1595:bool)  [unwired: 1 in, 5 out]
            n1621 = case shown="True" w1595 {
              frame False {
              }
              frame True {
                n1622 = Initialize Array(FALSE, 80 ("dimension size")) -> (w1601:bool[])
                n1623 = Array To Cluster(array=w1601) -> (cluster=w1597:T49)
                n1624 = local read "DecodeClust"() -> (w1600:T5)
                n1625 = Bundle By Name(cluster=w1600, "ClearEMG"=FALSE ("CtrlButtons.ResetTrial"), "KEMGClust"=w1597, "KEMGExtra"=dbl[] []) -> (w1599:T5)
                n1626 = local write "DecodeClust"(w1599) -> ()
              }
            }
          }
          event Value Change {
            n1627 = event-data() -> ("NewVal"=w1605:bool)  [unwired: 1 in, 5 out]
            n1628 = case shown="True" w1605 {
              frame False {
              }
              frame True {
                n1629 = Initialize Array(TRUE, 80 ("dimension size")) -> (w1610:bool[])
                n1630 = Array To Cluster(array=w1610) -> (cluster=w1606:T49)
                n1631 = local read "DecodeClust"() -> (w1607:T5)
                n1632 = Bundle By Name(cluster=w1607, "FillEMG"=FALSE ("CtrlButtons.ResetTrial"), "KEMGClust"=w1606) -> (w1608:T5)
                n1633 = local write "DecodeClust"(w1608) -> ()
              }
            }
          }
          event Value Change {
            n1634 = event-data() -> ()  [unwired: 1 in, 6 out]
            n1635 = local read "DecodeClust"() -> (w1628:T5)
            n1636 = Unbundle By Name(w1628) -> ("GainFill"=w1627:dbl, "ThreshFill"=w1626:dbl, "ModeFill"=w1617:T50, "SpdFill"=w1614:dbl)
            n1637 = Initialize Array(w1627, 12 ("dimension size"), 2 ("dimension size")) -> (w1632:dbl[][])
            n1638 = Initialize Array(w1626, 12 ("dimension size"), 2 ("dimension size")) -> (w1629:dbl[][])
            n1639 = Initialize Array(w1617, 12 ("dimension size")) -> (w1616:T43)
            n1640 = Initialize Array(w1614, 12 ("dimension size")) -> (w1613:dbl[])
            n1641 = Bundle By Name(cluster=w1628, "KMvntClust.KGain"=w1632, "KMvntClust.KThresh"=w1629, "KMvntClust.CtrlMode"=w1616, "KMvntClust.CtrlSpd"=w1613, "FillMvnts"=FALSE ("ClearKalman")) -> (w1619:T5)
            n1642 = Unbundle By Name(w1619) -> ("KMvntClust"=w1625:T46)
            n1643 = local write "DecodeClust"(w1619) -> ()
            n1644 = call "FeedbackDecode_KalmanMvnts2Str.vi"("KMvntClust"=w1625) -> ("KMvntStr"=w1622:string)
            n1645 = Concatenate Strings("UpdateKGainThresh:" ("string"), w1622) -> (w1621:string)
            n1646 = Bundle By Name(cluster=w1619, "EventStr"=w1621) -> (w1620:T5)
            n1647 = call "FeedbackDecode_MLComCtrl.vi"("DecodeClustIn"=w1620, "Mode"=T19."SendEvent") -> ()  [unwired: 6 in, 4 out]
          }
          event Value Change {
            n1648 = event-data() -> ("NewVal"=w1637:bool)  [unwired: 1 in, 5 out]
            n1649 = case shown="True" w1637 {
              frame False {
              }
              frame True {
                n1650 = Initialize Array(0.0 ("element"), 2 ("dimension size"), 12 ("dimension size")) -> (w1639:dbl[][])
                n1651 = local read "DecodeClust"() -> (w1642:T5)
                n1652 = Bundle By Name(cluster=w1642, "ClearTrials"=FALSE ("CtrlButtons.ResetTrial"), "TrialCnt"=w1639) -> (w1641:T5)
                n1653 = local write "DecodeClust"(w1641) -> ()
              }
            }
          }
          event Value Change {
            n1654 = event-data() -> ("NewVal"=w1652:dbl)  [unwired: 1 in, 5 out]
            n1655 = local read "LoopCnt"() -> (w1655:u64)
            n1656 = local read "NIPTime"() -> (w1650:dbl)
            n1657 = call-poly "FeedbackDecode_VariablesToString.vi"("ValueIn"=w1652, "FieldName"="Lag") -> ("StringOut"=w1662:string)  [unwired: 5 in]
            n1658 = local read "DecodeClust"() -> (w1660:T5)
            n1659 = Format Into String(w1655) -> (resulting string=w1646:string)  [unwired: 3 in, 1 out]
            n1660 = local read "EventParamsFID"() -> (w1659:refnum<file>)
            n1661 = call-poly "FeedbackDecode_VariablesToString.vi"("Format"="%0.0f", "ValueIn"=w1650, "FieldName"="NIPTime" ("Key Word")) -> ("StringOut"=w1647:string)  [unwired: 4 in]
            n1662 = Concatenate Strings("ChangeLag:SS.EventID=" ("string"), w1646) -> (w1654:string)
            n1663 = Concatenate Strings(w1654, ";", w1662, w1647) -> (w1653:string)
            n1664 = call "FeedbackDecode_WriteTextEOL.vi"("text"=w1653, "refnum in"=w1659) -> ()  [unwired: 8 in, 2 out]
            n1665 = Bundle By Name(cluster=w1660, "EventStr"=w1653) -> (w1651:T5)
            n1666 = call "FeedbackDecode_MLComCtrl.vi"("DecodeClustIn"=w1651, "Mode"=T19."SendEvent") -> ()  [unwired: 6 in, 4 out]
          }
          event Value Change {
            n1667 = event-data() -> ("NewVal"=w1670:dbl)  [unwired: 1 in, 5 out]
            n1668 = local read "LoopCnt"() -> (w1673:u64)
            n1669 = local read "NIPTime"() -> (w1668:dbl)
            n1670 = call-poly "FeedbackDecode_VariablesToString.vi"("ValueIn"=w1670, "FieldName"="KernelWidth") -> ("StringOut"=w1680:string)  [unwired: 5 in]
            n1671 = local read "DecodeClust"() -> (w1678:T5)
            n1672 = Format Into String(w1673) -> (resulting string=w1664:string)  [unwired: 3 in, 1 out]
            n1673 = local read "EventParamsFID"() -> (w1677:refnum<file>)
            n1674 = call-poly "FeedbackDecode_VariablesToString.vi"("Format"="%0.0f", "ValueIn"=w1668, "FieldName"="NIPTime" ("Key Word")) -> ("StringOut"=w1665:string)  [unwired: 4 in]
            n1675 = Concatenate Strings("ChangeKernel:SS.EventID=" ("string"), w1664) -> (w1672:string)
            n1676 = Concatenate Strings(w1672, ";", w1680, w1665) -> (w1671:string)
            n1677 = call "FeedbackDecode_WriteTextEOL.vi"("text"=w1671, "refnum in"=w1677) -> ()  [unwired: 8 in, 2 out]
            n1678 = Bundle By Name(cluster=w1678, "EventStr"=w1671) -> (w1669:T5)
            n1679 = call "FeedbackDecode_MLComCtrl.vi"("DecodeClustIn"=w1669, "Mode"=T19."SendEvent") -> ()  [unwired: 6 in, 4 out]
          }
          event Value Change {
            n1680 = event-data() -> ("NewVal"=w1688:dbl)  [unwired: 1 in, 5 out]
            n1681 = local read "LoopCnt"() -> (w1691:u64)
            n1682 = local read "NIPTime"() -> (w1686:dbl)
            n1683 = call-poly "FeedbackDecode_VariablesToString.vi"("ValueIn"=w1688, "FieldName"="TargRad") -> ("StringOut"=w1698:string)  [unwired: 5 in]
            n1684 = local read "DecodeClust"() -> (w1696:T5)
            n1685 = Format Into String(w1691) -> (resulting string=w1682:string)  [unwired: 3 in, 1 out]
            n1686 = local read "EventParamsFID"() -> (w1695:refnum<file>)
            n1687 = call-poly "FeedbackDecode_VariablesToString.vi"("Format"="%0.0f", "ValueIn"=w1686, "FieldName"="NIPTime" ("Key Word")) -> ("StringOut"=w1683:string)  [unwired: 4 in]
            n1688 = Concatenate Strings("ChangeTargRad:SS.EventID=" ("string"), w1682) -> (w1690:string)
            n1689 = Concatenate Strings(w1690, ";", w1698, w1683) -> (w1689:string)
            n1690 = call "FeedbackDecode_WriteTextEOL.vi"("text"=w1689, "refnum in"=w1695) -> ()  [unwired: 8 in, 2 out]
            n1691 = Bundle By Name(cluster=w1696, "EventStr"=w1689) -> (w1687:T5)
            n1692 = call "FeedbackDecode_MLComCtrl.vi"("DecodeClustIn"=w1687, "Mode"=T19."SendEvent") -> ()  [unwired: 6 in, 4 out]
          }
          event Value Change {
            n1693 = event-data() -> ("NewVal"=w1706:T37)  [unwired: 1 in, 5 out]
            n1694 = local read "LoopCnt"() -> (w1709:u64)
            n1695 = Format Into String(w1706) -> (resulting string=w1717:string)  [unwired: 3 in, 1 out]
            n1696 = local read "NIPTime"() -> (w1704:dbl)
            n1697 = local read "DecodeClust"() -> (w1714:T5)
            n1698 = Format Into String(w1709) -> (resulting string=w1700:string)  [unwired: 3 in, 1 out]
            n1699 = Concatenate Strings("SS.KinSrc='" ("string"), w1717, "';" ("string")) -> (w1718:string)
            n1700 = local read "EventParamsFID"() -> (w1713:refnum<file>)
            n1701 = call-poly "FeedbackDecode_VariablesToString.vi"("Format"="%0.0f", "ValueIn"=w1704, "FieldName"="NIPTime" ("Key Word")) -> ("StringOut"=w1701:string)  [unwired: 4 in]
            n1702 = Concatenate Strings("ChangeKinSrc:SS.EventID=" ("string"), w1700) -> (w1708:string)
            n1703 = Concatenate Strings(w1708, ";", w1718, w1701) -> (w1707:string)
            n1704 = call "FeedbackDecode_WriteTextEOL.vi"("text"=w1707, "refnum in"=w1713) -> ()  [unwired: 8 in, 2 out]
            n1705 = Bundle By Name(cluster=w1714, "EventStr"=w1707) -> (w1705:T5)
            n1706 = call "FeedbackDecode_MLComCtrl.vi"("DecodeClustIn"=w1705, "Mode"=T19."SendEvent") -> ()  [unwired: 6 in, 4 out]
          }
          event Value Change {
            n1707 = event-data() -> ("NewVal"=w1720:T23)  [unwired: 1 in, 5 out]
            n1708 = local read "LoopCnt"() -> (w1729:u64)
            n1709 = Format Into String(w1720) -> (resulting string=w1737:string)  [unwired: 3 in, 1 out]
            n1710 = local read "NIPTime"() -> (w1725:dbl)
            n1711 = local read "DecodeClust"() -> (w1734:T5)
            n1712 = Format Into String(w1729) -> (resulting string=w1721:string)  [unwired: 3 in, 1 out]
            n1713 = Concatenate Strings("SS.TestType='" ("string"), w1737, "';" ("string")) -> (w1738:string)
            n1714 = local read "EventParamsFID"() -> (w1733:refnum<file>)
            n1715 = call-poly "FeedbackDecode_VariablesToString.vi"("Format"="%0.0f", "ValueIn"=w1725, "FieldName"="NIPTime" ("Key Word")) -> ("StringOut"=w1722:string)  [unwired: 4 in]
            n1716 = Concatenate Strings("ChangeTestType:SS.EventID=" ("string"), w1721) -> (w1728:string)
            n1717 = Concatenate Strings(w1728, ";", w1738, w1722) -> (w1727:string)
            n1718 = call "FeedbackDecode_WriteTextEOL.vi"("text"=w1727, "refnum in"=w1733) -> ()  [unwired: 8 in, 2 out]
            n1719 = Bundle By Name(cluster=w1734, "EventStr"=w1727) -> (w1726:T5)
            n1720 = call "FeedbackDecode_MLComCtrl.vi"("DecodeClustIn"=w1726, "Mode"=T19."SendEvent") -> ()  [unwired: 6 in, 4 out]
          }
          event Value Change {
            n1721 = event-data() -> ("NewVal"=w1740:bool)  [unwired: 1 in, 5 out]
            n1722 = case shown="True" w1740 {
              frame False {
              }
              frame True {
                n1723 = local read "LoopCnt"() -> (w1753:u64)
                n1724 = local read "NIPTime"() -> (w1746:dbl)
                n1725 = Format Into String(w1753) -> (resulting string=w1742:string)  [unwired: 3 in, 1 out]
                n1726 = local read "EventParamsFID"() -> (w1757:refnum<file>)
                n1727 = call-poly "FeedbackDecode_VariablesToString.vi"("Format"="%0.0f", "ValueIn"=w1746, "FieldName"="NIPTime" ("Key Word")) -> ("StringOut"=w1743:string)  [unwired: 4 in]
                n1728 = Concatenate Strings("ResetVRE:SS.EventID=" ("string"), w1742) -> (w1752:string)
                n1729 = Concatenate Strings(w1752, ";", w1743) -> (w1751:string)
                n1730 = local read "DecodeClust"() -> (w1758:T5)
                n1731 = call "FeedbackDecode_WriteTextEOL.vi"("text"=w1751, "refnum in"=w1757) -> ()  [unwired: 8 in, 2 out]
                n1732 = Bundle By Name(cluster=w1758, "EventStr"=w1751, "CtrlButtons.ResetVRE"=FALSE ("ResetVRE")) -> (w1750:T5)
                n1733 = property on="StimMode" class="Enum (strict)"("Val(Sgnl)"=enum16{"Off", "Manual", "MSMS", "VRE"}."Off" ("Value (Signaling)")) -> ()  [unwired: 2 in, 2 out]
                n1734 = call "FeedbackDecode_MLComCtrl.vi"("DecodeClustIn"=w1750, "Mode"=T19."SendEvent") -> ("DecodeClustOut"=w1748:T5)  [unwired: 6 in, 3 out]
                n1735 = local write "DecodeClust"(w1748) -> ()
              }
            }
          }
          event Value Change {
            n1736 = event-data() -> ("NewVal"=w1759:bool)  [unwired: 1 in, 5 out]
            n1737 = case shown="True" w1759 {
              frame False {
              }
              frame True {
                n1738 = local read "LoopCnt"() -> (w1772:u64)
                n1739 = local read "NIPTime"() -> (w1765:dbl)
                n1740 = Format Into String(w1772) -> (resulting string=w1761:string)  [unwired: 3 in, 1 out]
                n1741 = local read "EventParamsFID"() -> (w1776:refnum<file>)
                n1742 = Concatenate Strings("StopVRE:SS.EventID=" ("string"), w1761) -> (w1771:string)
                n1743 = call-poly "FeedbackDecode_VariablesToString.vi"("Format"="%0.0f", "ValueIn"=w1765, "FieldName"="NIPTime" ("Key Word")) -> ("StringOut"=w1762:string)  [unwired: 4 in]
                n1744 = Concatenate Strings(w1771, ";", w1762) -> (w1770:string)
                n1745 = local read "DecodeClust"() -> (w1777:T5)
                n1746 = call "FeedbackDecode_WriteTextEOL.vi"("text"=w1770, "refnum in"=w1776) -> ()  [unwired: 8 in, 2 out]
                n1747 = Bundle By Name(cluster=w1777, "EventStr"=w1770, "CtrlButtons.StopVRE"=FALSE ("ResetVRE")) -> (w1769:T5)
                n1748 = property on="StimMode" class="Enum (strict)"("Val(Sgnl)"=enum16{"Off", "Manual", "MSMS", "VRE"}."Off" ("Value (Signaling)")) -> ()  [unwired: 2 in, 2 out]
                n1749 = call "FeedbackDecode_MLComCtrl.vi"("DecodeClustIn"=w1769, "Mode"=T19."SendEvent") -> ("DecodeClustOut"=w1767:T5)  [unwired: 6 in, 3 out]
                n1750 = local write "DecodeClust"(w1767) -> ()
              }
            }
          }
          event Value Change {
            n1751 = event-data() -> ("NewVal"=w1778:bool)  [unwired: 1 in, 5 out]
            n1752 = case shown="True" w1778 {
              frame False {
              }
              frame True {
                n1753 = local read "LoopCnt"() -> (w1790:u64)
                n1754 = local read "NIPTime"() -> (w1784:dbl)
                n1755 = Format Into String(w1790) -> (resulting string=w1780:string)  [unwired: 3 in, 1 out]
                n1756 = local read "EventParamsFID"() -> (w1794:refnum<file>)
                n1757 = Concatenate Strings("ConARD:SS.EventID=" ("string"), w1780) -> (w1789:string)
                n1758 = call-poly "FeedbackDecode_VariablesToString.vi"("Format"="%0.0f", "ValueIn"=w1784, "FieldName"="NIPTime" ("Key Word")) -> ("StringOut"=w1781:string)  [unwired: 4 in]
                n1759 = Concatenate Strings(w1789, ";", w1781) -> (w1788:string)
                n1760 = local read "DecodeClust"() -> (w1795:T5)
                n1761 = call "FeedbackDecode_WriteTextEOL.vi"("text"=w1788, "refnum in"=w1794) -> ()  [unwired: 8 in, 2 out]
                n1762 = Bundle By Name(cluster=w1795, "EventStr"=w1788, "CtrlButtons.ConARD"=FALSE ("ResetVRE")) -> (w1787:T5)
                n1763 = call "FeedbackDecode_MLComCtrl.vi"("DecodeClustIn"=w1787, "Mode"=T19."SendEvent") -> ("DecodeClustOut"=w1785:T5)  [unwired: 6 in, 3 out]
                n1764 = local write "DecodeClust"(w1785) -> ()
              }
            }
          }
          event Value Change {
            n1765 = event-data() -> ("NewVal"=w1797:bool)  [unwired: 1 in, 4 out]
            n1766 = case shown="True" w1797 {
              frame False {
              }
              frame True {
                n1767 = property on="MvntList" class="Arr (strict)"() -> ("Index Values"=w1801:u32[])  [unwired: 2 in, 2 out]
                n1768 = local read "MvntBuilder"() -> (w1805:T6)
                n1769 = Index Array(array=w1801) -> (element=w1806:u32)  [unwired: 1 in]
                n1770 = local read "DecodeClust"() -> (w1800:T5)
                n1771 = Bundle By Name(cluster=w1800, "CtrlButtons.StartTrials"=FALSE) -> (w1798:T5)
                n1772 = call "FeedbackDecode_SetMvntBuilder.vi"("MvntBuilderIn"=w1805, "MvntIdx"=w1806) -> ("MvntBuilderOut"=w1804:T6)  [unwired: 1 in]
                n1773 = Bundle By Name(cluster=w1804, "Set"=FALSE) -> (w1802:T6)
                n1774 = local write "MvntBuilder"(w1802) -> ()
                n1775 = local write "DecodeClust"(w1798) -> ()
              }
            }
          }
          event Value Change {
            n1776 = event-data() -> ("NewVal"=w1808:bool)  [unwired: 1 in, 4 out]
            n1777 = case shown="True" w1808 {
              frame False {
              }
              frame True {
                n1778 = local read "MvntBuilder"() -> (w1813:T6)
                n1779 = local read "DecodeClust"() -> (w1812:T5)
                n1780 = Bundle By Name(cluster=w1812, "CtrlButtons.StartTrials"=FALSE) -> (w1810:T5)
                n1781 = Bundle By Name(cluster=w1813, "MvntList"=T24 [], "Clear"=FALSE ("Set")) -> (w1814:T6)
                n1782 = local write "MvntBuilder"(w1814) -> ()
                n1783 = local write "DecodeClust"(w1810) -> ()
              }
            }
          }
          event Value Change {
            n1784 = event-data() -> ("NewVal"=w1817:bool)  [unwired: 1 in, 5 out]
            n1785 = case shown="True" w1817 {
              frame False {
              }
              frame True {
                n1786 = flat-sequence {
                  frame #0 {
                    n1787 = local read "MvntBuilder"() -> (w1821:T6)
                    n1788 = local read "DecodeClust"() -> (w1820:T5)
                    n1789 = Bundle By Name(cluster=w1820, "CtrlButtons.StartTrials"=FALSE) -> (w1818:T5)
                    n1790 = Bundle By Name(cluster=w1821, "Load"=FALSE ("Set")) -> (w1822:T6)
                    n1791 = local write "MvntBuilder"(w1822) -> ()
                    n1792 = local write "DecodeClust"(w1818) -> ()
                  }
                  frame #1 {
                    n1793 = local read "MvntBuilder"() -> (w1825:T6)
                    n1794 = call "FeedbackDecode_MvntListIO.vi"("MvntBuilderIn"=w1825, "Mode"=enum16{"Read", "Write"}."Read") -> ("MvntBuilderOut"=w1824:T6)  [unwired: 1 in]
                    n1795 = Unbundle By Name(w1824) -> ("MvntList"=w1827:T24)
                    n1796 = property on="MvntList" class="Arr (strict)"("Val(Sgnl)"=w1827) -> ()  [unwired: 2 in, 2 out]
                  }
                }
              }
            }
          }
          event Value Change {
            n1797 = event-data() -> ("NewVal"=w1828:bool)  [unwired: 1 in, 5 out]
            n1798 = case shown="True" w1828 {
              frame False {
              }
              frame True {
                n1799 = flat-sequence {
                  frame #0 {
                    n1800 = local read "MvntBuilder"() -> (w1833:T6)
                    n1801 = local read "DecodeClust"() -> (w1832:T5)
                    n1802 = Bundle By Name(cluster=w1832, "CtrlButtons.StartTrials"=FALSE) -> (w1830:T5)
                    n1803 = Bundle By Name(cluster=w1833, "Save"=FALSE ("Set")) -> (w1834:T6)
                    n1804 = local write "MvntBuilder"(w1834) -> ()
                    n1805 = local write "DecodeClust"(w1830) -> ()
                  }
                  frame #1 {
                    n1806 = local read "MvntBuilder"() -> (w1836:T6)
                    n1807 = call "FeedbackDecode_MvntListIO.vi"("MvntBuilderIn"=w1836, "Mode"=enum16{"Read", "Write"}."Write") -> ()  [unwired: 1 in, 1 out]
                  }
                }
              }
            }
          }
          event Value Change {
            n1808 = event-data() -> ("OldVal"=w1841:T24, "NewVal"=w1840:T24)  [unwired: 1 in, 4 out]
            n1809 = Array Size(array=w1841) -> (size(s)=w1842:i32)
            n1810 = Array Size(array=w1840) -> (size(s)=w1843:i32)
            n1811 = Not Equal?(x=w1842, y=w1843) -> (x != y?=w1839:bool)
            n1812 = case shown="True" w1839 {
              frame False {
              }
              frame True {
                n1813 = local read "MvntBuilder"() -> (w1846:T6)
                n1814 = local read "DecodeClust"() -> (w1856:T5)
                n1815 = Bundle By Name(cluster=w1856, "CtrlButtons.StartTrials"=FALSE) -> (w1854:T5)
                n1816 = Unbundle By Name(w1846) -> ("Mode"=w1853:enum16{"Selected", "Block", "Random"}, "NTrials"=w1850:dbl, "MvntList"=w1849:T24)
                n1817 = property on="MvntList" class="Arr (strict)"() -> ("Index Values"=w1847:u32[])  [unwired: 2 in, 2 out]
                n1818 = Array Size(array=w1849) -> (size(s)=w1848:i32)
                n1819 = Index Array(array=w1847) -> (element=w1851:u32)  [unwired: 1 in]
                n1820 = local write "DecodeClust"(w1854) -> ()
                n1821 = call "FeedbackDecode_GenRandBlockIdxs2.vi"("Mode"=w1853, "Reset"=TRUE, "NumTrials"=w1850, "NumIdxs"=w1848, "CurrIdx"=w1851) -> ("Perc"=w1845:dbl)  [unwired: 1 out]
                n1822 = Bundle By Name(cluster=w1846, "PercTrials"=w1845) -> (w1844:T6)
                n1823 = local write "MvntBuilder"(w1844) -> ()
              }
            }
          }
          event Value Change {
            n1824 = event-data() -> ("NewVal"=w1857:dbl)  [unwired: 1 in, 5 out]
            n1825 = local read "MSMSSphere"() -> (w1863:dbl[][])
            n1826 = Initialize Array(w1857, 6 ("dimension size")) -> (w1859:dbl[])
            n1827 = property on="TargRad" class="DigNum (strict)"("Val(Sgnl)"=w1857) -> ()  [unwired: 2 in, 2 out]
            n1828 = Replace Array Subset(array=w1863, new element=w1859, index (col)=3 ("disabled index (col)")) -> (w1862:dbl[][])  [unwired: 1 in]
            n1829 = local write "MSMSSphere"(w1862) -> ()
          }
          event User Event {
            n1830 = event-data() -> ("MvntEvnt"=w1865:dbl)  [unwired: 1 in, 4 out]
            n1831 = Build Array(w1865) -> (w1864:dbl[])
            n1832 = property on="MvntList" class="Arr (strict)"("Index Values"=w1864) -> ()  [unwired: 2 in, 2 out]
          }
          event "MedianHM": Mouse Down {
            w1876 = cluster{"X":i32, "Y":i32} {"X"=0, "Y"=0} ("MousePos")
            w1877 = enum16{"Initialize", "Run", "Mouse"}."Mouse" ("Mode")
            n1833 = event-data() -> ("PlatMods"=w1871:T51, "Coords"=w1874:T45)  [unwired: 1 in, 4 out]
            n1834 = Cluster To Array(cluster=w1871) -> (array=w1870:bool[])
            n1835 = Boolean Array To Number(Boolean array=w1870) -> (number=w1869:u32)
            n1836 = local read "DecodeClust"() -> (w1873:T5)
            n1837 = local read "UEAHMIdx"() -> (w1890:i32[])
            n1838 = call "FeedbackDecode_PlotHeatmap.vi"("MousePos"=w1874, "Instance"=0, "Mode"=w1877) -> ("CurrPos"=w1889:i32)  [unwired: 3 in, 1 out]
            n1839 = call "FeedbackDecode_PlotHeatmap.vi"("MousePos"=w1876, "Instance"=1, "Mode"=w1877) -> ()  [unwired: 3 in, 2 out]
            n1840 = call "FeedbackDecode_PlotHeatmap.vi"("MousePos"=w1876, "Instance"=2, "Mode"=w1877) -> ()  [unwired: 3 in, 2 out]
            n1841 = Search 1D Array(1D array=w1890, element=w1889) -> (index of element=w1888:i32)  [unwired: 1 in]
            n1842 = Increment(x=w1888) -> (x+1=w1875:i32)
            n1843 = case shown="4" w1869 {
              tunnel: w1875 -> [_ w1894 w1898]
              tunnel: w1873 -> [w1891 w1893 w1897]
              tunnel: [w1891 w1892 w1896] -> w1872
              frame 0, Default {
              }
              frame 18 {
                # "ctrl"
                n1844 = call "FeedbackDecode_UpdateDecodeClustElect.vi"("DecodeClustIn"=w1893, "KalmanElect"=w1894) -> ("DecodeClustOut"=w1892:T5)  [unwired: 1 in]
              }
              frame 4 {
                # "alt"
                n1845 = Unbundle By Name(w1897) -> ("BadUEAElects"=w1899:dbl[])
                n1846 = Insert Into Array(array=w1899, new element=w1898) -> (w1895:dbl[])  [unwired: 1 in]
                n1847 = Bundle By Name(cluster=w1897, "BadUEAElects"=w1895) -> (w1896:T5)
                n1848 = property on="BadUEAElects" class="Arr (strict)"("Val(Sgnl)"=w1895) -> ()  [unwired: 2 in, 2 out]
              }
            }
            n1849 = local read "LoopCnt"() -> (w1882:u64)
            n1850 = call-poly "FeedbackDecode_VariablesToString.vi"("Format"="%0.0f", "ValueIn"=w1875, "FieldName"="SelElect") -> ("StringOut"=w1884:string)  [unwired: 4 in]
            n1851 = local write "SelElect"(w1875) -> ()
            n1852 = local write "BaseCnt2"(w1882) -> ()
            n1853 = Bundle By Name(cluster=w1872, "ClearWfs"=TRUE, "SelElect"=w1875, "EventStr"=w1884) -> (w1868:T5)
            n1854 = call "FeedbackDecode_MLComCtrl.vi"("DecodeClustIn"=w1868, "Mode"=T19."SendEvent") -> ("DecodeClustOut"=w1867:T5)  [unwired: 6 in, 3 out]
            n1855 = local write "DecodeClust"(w1867) -> ()
          }
          event "UlnarHM": Mouse Down {
            w1911 = cluster{"X":i32, "Y":i32} {"X"=0, "Y"=0} ("MousePos")
            w1912 = enum16{"Initialize", "Run", "Mouse"}."Mouse" ("Mode")
            n1856 = event-data() -> ("PlatMods"=w1907:T51, "Coords"=w1910:T45)  [unwired: 1 in, 4 out]
